vi "Create from SCP Receive.vi"(8 "Error In":errorcluster, 9 "Remote Source Path":string, 10 "File Info In":refnum<class "File Info.lvclass">, 11 "Session":refnum<class "Session.lvclass">) -> (0 "Error Out":errorcluster, 2 "File Info Out":refnum<class "File Info.lvclass">, 3 "Channel":refnum<class "Channel.lvclass">)   [LabVIEW 2018, in "Toolkit.lvlib" / "Channel.lvclass"]
uses:
  Channel.lvclass
  Session/Session.lvclass
  File Info/File Info.lvclass
  File Info/File Info.lvclass/File Info.ctl
  Session/Session.lvclass/Session.ctl
  SSH/SSH.lvclass/SSH.ctl
  Channel.lvclass/Channel.ctl
  Toolkit.lvlib
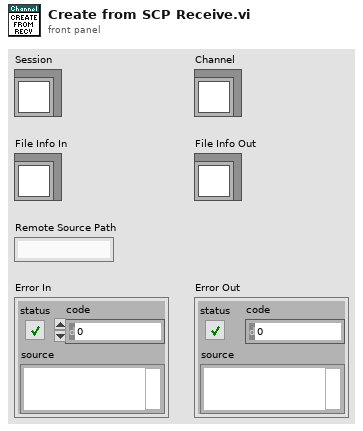
[diagram p1: front panel]
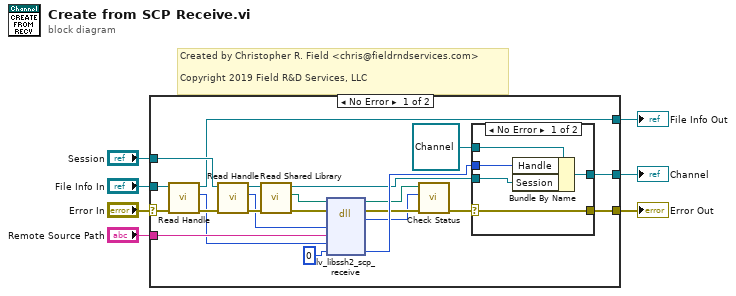
[diagram p0: block diagram]
diagram:
  # "Created by Christopher R. Field <chris@fieldrndservices.com>\n\nCopyright 2019 Field R&D Services, LLC"
  n1 = case shown="No Error" "Error In" {
    selector: "Error In" -> [w12 w38]
    tunnel: [w27 w38] -> w6
    tunnel: "Session" -> [w28 _]
    tunnel: [w29 _] -> w4
    tunnel: "Remote Source Path" -> [w13 _]
    tunnel: "File Info In" -> [w10 w37]
    tunnel: [w8 w37] -> w1
    frame No Error {
      n2 = call "Read Handle.vi"("Error In"=w12, "File Info In"=w10) -> ("Error Out"=w11:errorcluster, "Handle"=w9:u64, "File Info Out"=w8:refnum<class "File Info.lvclass">)  [unwired: 7 in]
      n3 = call "Read Handle.vi"("Error In"=w11, "Session In"=w28) -> ("Erorr Out"=w24:errorcluster, "Handle"=w21:u64, "Session Out"=w25:refnum<class "Session.lvclass">)  [unwired: 7 in]
      n4 = call "Read Shared Library.vi"("Error In"=w24, "Session In"=w25) -> ("Erorr Out"=w23:errorcluster, "libssh2lv Shared Library"=w22:path, "Session Out"=w14:refnum<class "Session.lvclass">)  [unwired: 7 in]
      n5 = dll-call lib="libssh2lv.*" fn="lv_libssh2_scp_receive"(path in=w22, error in=w23, "session"=w21, "path"=w13, "file_info"=w9, "handle"=u64 0) -> (path out=w16:path, error out=w18:errorcluster, "status"=w17:i32, "handle"=w19:u64)  [unwired: 4 in]
      n6 = call "Check Status.vi"("Error In"=w18, "Status"=w17, "libssh2lv Shared Library In"=w16) -> ("Error Out"=w15:errorcluster)  [unwired: 7 in, 1 out]
      n7 = case shown="No Error" w15 {
        selector: w15 -> [w33 w36]
        tunnel: [w30 w35] -> w29
        tunnel: w19 -> [w34 _]
        tunnel: [w33 w36] -> w27
        tunnel: w14 -> [w32 _]
        tunnel: refnum<class "Channel.lvclass"> refnum ("Toolkit.lvlib:Channel.lvclass") -> [w31 w35]
        frame No Error {
          n8 = Bundle By Name(cluster=w31, "Handle"=w34, "Session"=w32) -> (w30:refnum<class "Channel.lvclass">)
        }
        frame Error {
        }
      }
    }
    frame Error {
    }
  }
  "Error Out" <- w6
  "Channel" <- w4
  "File Info Out" <- w1
